vi "PH_VacuumControl.Search Device.vi"(0 "i ref in":refnum<vi>, 5 "error in (no error)":errorcluster) -> (14 "i ref out":refnum<vi>, 17 "Device found":bool, 19 "error out":errorcluster)   [LabVIEW 2014, in "PH_VacuumControl.lvlib"]
doc: "This VI searches for the device which is given by a firmware number. It is indicated if this is found succesfully, and connection data are written wo own attributes."
uses:
  PH_VacuumControl.lvlib
  instr.lib/AGCxxx/AGCxxx/AGCxxx VISA Control.ctl
  instr.lib/AGCxxx/AGCxxx - Driver.lvlib
  PH_Common/PH_Common.lvlib
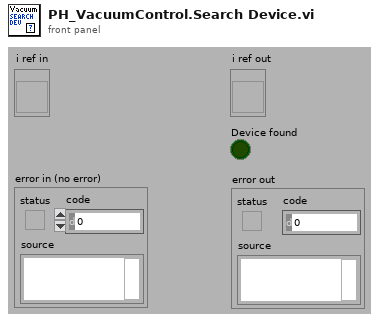
[diagram p1: front panel]
types:
  T1 = typedef "PH_VacuumControl.lvlib/PH_VacuumControl.i attribute.ctl" = cluster{"GUI Refs":cluster{"Exit":refnum<vi>, "Set Unit":refnum<vi>, "Device found":refnum<vi>, "Busy":refnum<vi>, "State":refnum<vi>, "Delete":refnum<vi>, "Channels":refnum<vi>, "Channel Name":refnum<vi>, "Trend":refnum<vi>, "Logarithmic":refnum<vi>, "Limit reached":refnum<vi>, "Channel Name 1 MT":refnum<vi>, "Channel Name 2 MT":refnum<vi>, "Trend MT":refnum<vi>, "Logarithmic MT":refnum<vi>, "Limit reached MT":refnum<vi>}, "Device found":bool, "Busy":bool, "Selected Unit":i32, "Channels [mbar]":T2, "Channel Names":cluster{"Channel 1":string, "Channel 2":string, "Channel 3":string, "Channel 4":string, "Channel 5":string, "Channel 6":string}, "Status":T3, "AGCxxx VISA Cluster":T4, "Instr Firmware Revision":string, "Service IDs Pressure":cluster{"Channel 1":i32, "Channel 2":i32, "Channel 3":i32, "Channel 4":i32, "Channel 5":i32, "Channel 6":i32}, "Service IDs Limits":cluster{"Channel 1":i32, "Channel 2":i32, "Channel 3":i32, "Channel 4":i32, "Channel 5":i32, "Channel 6":i32}, "Trend":cluster{"Start Point":timestamp, "Pressures [mbar] Channel 1":dbl[], "Pressures [mbar] Channel 2":dbl[], "Pressures [mbar] Channel 3":dbl[], "Pressures [mbar] Channel 4":dbl[], "Pressures [mbar] Channel 5":dbl[], "Pressures [mbar] Channel 6":dbl[], "Timebase [s]":i32[], "Trend Channel":u16, "Start Fit":dbl, "Trend Channel 1 MT":u16, "Trend Channel 2 MT":u16, "Start or continue Fit MT":dbl, "Continue or start Fit MT":dbl, "Datasets strored":i32, "Dataarray Size":i32}, "Running":bool}
  T2 = typedef "PH_VacuumControl.lvlib/PH_VacuumControl.Channels.ctl" = cluster{"Channel 1":dbl, "Channel 2":dbl, "Channel 3":dbl, "Channel 4":dbl, "Channel 5":dbl, "Channel 6":dbl, "Name Channel 1":string, "Name Channel 2":string, "Name Channel 3":string, "Name Channel 4":string, "Name Channel 5":string, "Name Channel 6":string, "Upper Limit":dbl, "Upper Limit 2":dbl, "Upper Limit 3":dbl, "Upper Limit 4":dbl, "Upper Limit 5":dbl, "Upper Limit 6":dbl}
  T3 = typedef "PH_StatusHandler.lvlib/PH_StatusHandler.Status.ctl" = i16
  T4 = typedef "AGCxxx - Driver.lvlib/AGCxxx VISA Control.ctl" = cluster{"VISA resource name":refnum<visa-resource-name>, "VISA Timeout Value (1000 ms)":u32, "Lock Timeout (1000 ms)":u32, "MAX Channel (6)":i32}
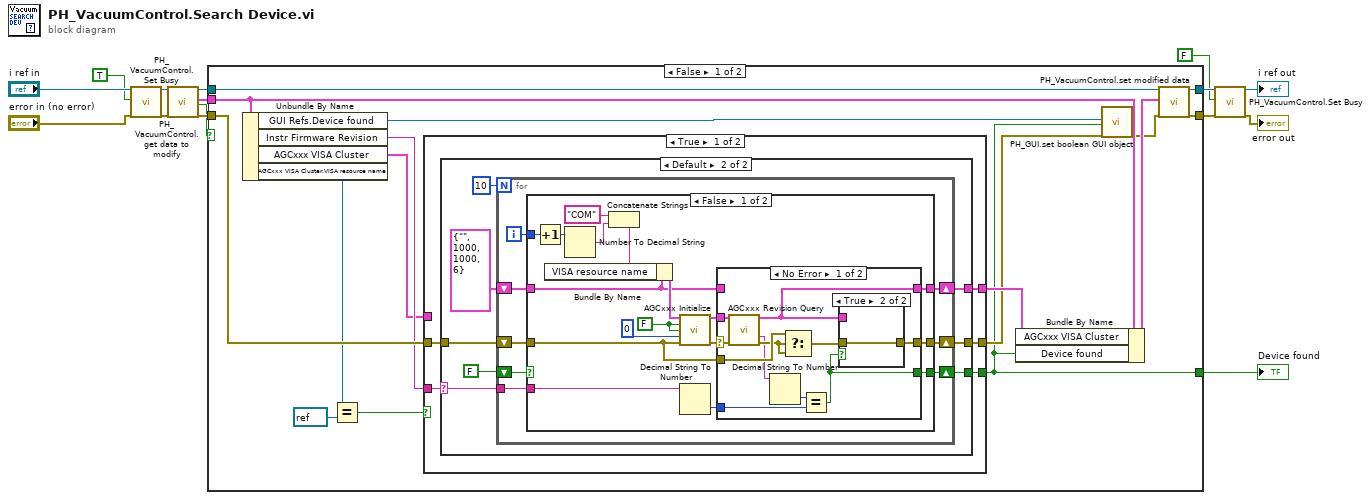
[diagram p0: block diagram]
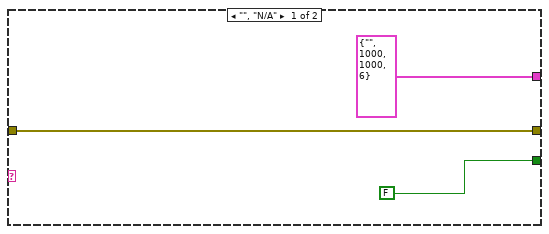
[diagram p2: hidden frame]
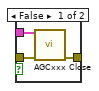
[diagram p3: hidden frame]
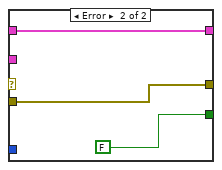
[diagram p4: hidden frame]
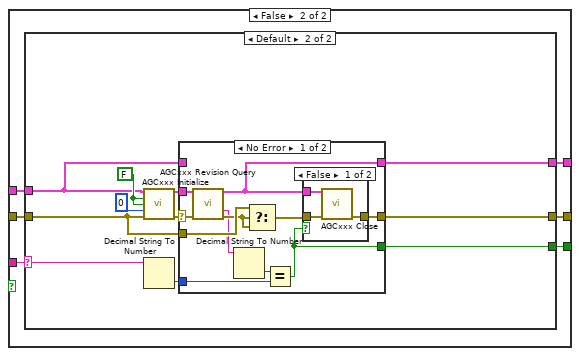
[diagram p6: hidden frame]
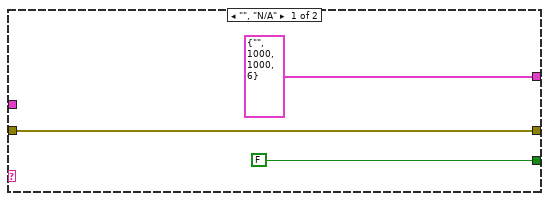
[diagram p7: hidden frame]
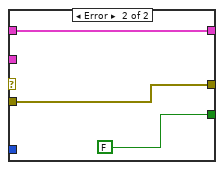
[diagram p9: hidden frame]
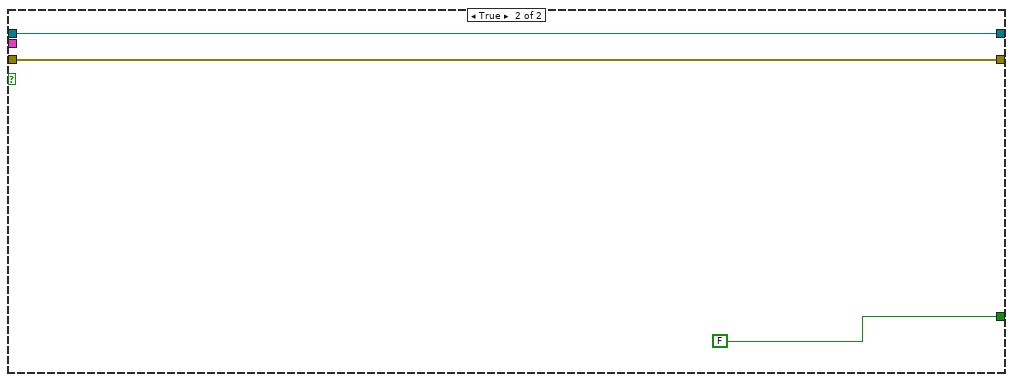
[diagram p10: hidden frame]
diagram:
  n1 = call "PH_VacuumControl.Set Busy.vi"("i ref in"="i ref in", "Busy"=TRUE, "error in (no error)"="error in (no error)") -> ("i ref out"=w7:refnum<vi>, "error out"=w9:errorcluster)  [unwired: 14 in, 1 out]
  n2 = call "PH_VacuumControl.get data to modify.vi"("i ref in"=w7, "error in (no error)"=w9) -> ("i ref out"=w14:refnum<vi>, "i attribute"=w13:T1, "timed out"=w12:bool, "error out"=w15:errorcluster)  [unwired: 14 in]
  n3 = case shown="False" w12 {
    tunnel: w15 -> [w31 w133]
    tunnel: w14 -> [w29 w134]
    tunnel: w13 -> [w28 _]
    tunnel: [w26 w133] -> w4
    tunnel: [w24 w134] -> w2
    tunnel: [w20 FALSE] -> w11
    frame False {
      n4 = Unbundle By Name(w28) -> ("GUI Refs.Device found"=w23:refnum<vi>, "Instr Firmware Revision"=w30:string, "AGCxxx VISA Cluster"=w16:T4, "AGCxxx VISA Cluster.VISA resource name"=w19:refnum<visa-resource-name>)
      n5 = Equal?(x=w19, y=refnum<visa-resource-name> refnum ("AGCxxx VISA Cluster.VISA resource name")) -> (x = y?=w17:bool)
      n6 = case shown="True" w17 {
        tunnel: w31 -> [w36 w99]
        tunnel: w30 -> [w35 w98]
        tunnel: [w34 w97] -> w27
        tunnel: [w33 w96] -> w22
        tunnel: [w32 w95] -> w20
        tunnel: w16 -> [_ w94]
        frame True {
          n7 = case shown="Default" w35 {
            selector: w35 -> [_ w43]
            tunnel: [FALSE w47] -> w32
            tunnel: [T4 {"VISA resource name"="", "VISA Timeout Value (1000 ms)"=1000, "Lock Timeout (1000 ms)"=1000, "MAX Channel (6)"=6} ("dup AGCxxx VISA Cluster") w46] -> w34
            tunnel: [w39 w45] -> w33
            tunnel: w36 -> [w39 w44]
            frame "", "N/A" {
            }
            frame Default {
              n8 = for {
                N: 10 -> [_]
                tunnel: w43 -> [w51]
                shift-right: [w53] -> w45
                shift-left: w44 -> [w52]
                shift-right: [w55] -> w47
                shift-left: FALSE -> [w49]
                shift-right: [w54] -> w46
                shift-left: T4 {"VISA resource name"="", "VISA Timeout Value (1000 ms)"=1000, "Lock Timeout (1000 ms)"=1000, "MAX Channel (6)"=6} ("dup AGCxxx VISA Cluster") -> [w48]
                i -> [w50]
                n9 = case shown="False" w49 {
                  selector: w49 -> [_ w91]
                  tunnel: [w71 w91] -> w55
                  tunnel: [w70 w93] -> w54
                  tunnel: [w69 w92] -> w53
                  tunnel: w52 -> [w59 w92]
                  tunnel: w51 -> [w57 _]
                  tunnel: w50 -> [w63 _]
                  tunnel: w48 -> [w58 w93]
                  frame False {
                    w66 = FALSE ("ID Query (T: Check)")
                    n10 = Increment(x=w63) -> (x+1=w62:i32)
                    n11 = Number To Decimal String(number=w62) -> (decimal integer string=w61:string)  [unwired: 1 in]
                    n12 = Concatenate Strings("COM", w61) -> (w64:string)
                    n13 = Bundle By Name(cluster=w58, "VISA resource name"=w64) -> (w72:T4)
                    n14 = call "AGCxxx Initialize.vi"("AGCxxx VISA Cluster"=w72, "ID Query (T: Check)"=w66, "Reset (T: Reset)"=w66, "access mode"=u32 0, "error in (no error)"=w59) -> ("dup AGCxxx VISA Cluster"=w68:T4, "error out"=w60:errorcluster)  [unwired: 9 in]
                    n15 = Decimal String To Number(string=w57) -> (number=w56:i32)  [unwired: 2 in, 1 out]
                    n16 = case shown="No Error" w60 {
                      selector: w60 -> [w78 _]
                      tunnel: [w83 FALSE] -> w71
                      tunnel: [w82 w89] -> w70
                      tunnel: [w81 w90] -> w69
                      tunnel: w68 -> [w80 _]
                      tunnel: w56 -> [w79 _]
                      tunnel: w59 -> [w76 w90]
                      tunnel: w58 -> [_ w89]
                      frame No Error {
                        n17 = call "AGCxxx Revision Query.vi"("AGCxxx VISA Cluster"=w80, "error in (no error)"=w78) -> ("dup AGCxxx VISA Cluster"=w82:T4, "Instr Firmware Revision"=w74:string, "error out"=w75:errorcluster)  [unwired: 10 in, 1 out]
                        n18 = Decimal String To Number(string=w74) -> (number=w73:i32)  [unwired: 2 in, 1 out]
                        n19 = Select(t=w76, s=w75, f=w75) -> (s? t:f=w77:errorcluster)
                        n20 = Equal?(x=w73, y=w79) -> (x = y?=w83:bool)
                        n21 = case shown="True" w83 {
                          tunnel: [w86 w87] -> w81
                          tunnel: w82 -> [w85 _]
                          tunnel: w77 -> [w84 w87]
                          frame False {
                            n22 = call "AGCxxx Close.vi"("AGCxxx VISA Cluster"=w85, "error in (no error)"=w84) -> ("error out"=w86:errorcluster)  [unwired: 13 in]
                          }
                          frame True {
                          }
                        }
                      }
                      frame Error {
                      }
                    }
                  }
                  frame True {
                  }
                }
              }
            }
          }
        }
        frame False {
          n23 = case shown="Default" w98 {
            selector: w98 -> [_ w109]
            tunnel: [FALSE w113] -> w95
            tunnel: [T4 {"VISA resource name"="", "VISA Timeout Value (1000 ms)"=1000, "Lock Timeout (1000 ms)"=1000, "MAX Channel (6)"=6} ("dup AGCxxx VISA Cluster") w112] -> w97
            tunnel: [w102 w111] -> w96
            tunnel: w99 -> [w102 w110]
            tunnel: w94 -> [_ w103]
            frame "", "N/A" {
            }
            frame Default {
              w106 = FALSE ("ID Query (T: Check)")
              n24 = call "AGCxxx Initialize.vi"("AGCxxx VISA Cluster"=w103, "ID Query (T: Check)"=w106, "Reset (T: Reset)"=w106, "access mode"=u32 0, "error in (no error)"=w110) -> ("dup AGCxxx VISA Cluster"=w108:T4, "error out"=w105:errorcluster)  [unwired: 9 in]
              n25 = Decimal String To Number(string=w109) -> (number=w104:i32)  [unwired: 2 in, 1 out]
              n26 = case shown="No Error" w105 {
                selector: w105 -> [w119 _]
                tunnel: [w124 FALSE] -> w113
                tunnel: [w123 w129] -> w112
                tunnel: [w122 w131] -> w111
                tunnel: w108 -> [w121 _]
                tunnel: w104 -> [w120 _]
                tunnel: w110 -> [w117 w131]
                tunnel: w103 -> [_ w129]
                frame No Error {
                  n27 = call "AGCxxx Revision Query.vi"("AGCxxx VISA Cluster"=w121, "error in (no error)"=w119) -> ("dup AGCxxx VISA Cluster"=w123:T4, "Instr Firmware Revision"=w115:string, "error out"=w116:errorcluster)  [unwired: 10 in, 1 out]
                  n28 = Decimal String To Number(string=w115) -> (number=w114:i32)  [unwired: 2 in, 1 out]
                  n29 = Select(t=w117, s=w116, f=w116) -> (s? t:f=w118:errorcluster)
                  n30 = Equal?(x=w114, y=w120) -> (x = y?=w124:bool)
                  n31 = case shown="False" w124 {
                    tunnel: [w127 w128] -> w122
                    tunnel: w123 -> [w126 _]
                    tunnel: w118 -> [w125 w128]
                    frame False {
                      n32 = call "AGCxxx Close.vi"("AGCxxx VISA Cluster"=w126, "error in (no error)"=w125) -> ("error out"=w127:errorcluster)  [unwired: 13 in]
                    }
                    frame True {
                    }
                  }
                }
                frame Error {
                }
              }
            }
          }
        }
      }
      n33 = Bundle By Name(cluster=w28, "AGCxxx VISA Cluster"=w27, "Device found"=w20) -> (w25:T1)
      n34 = call "PH_GUI.set boolean GUI object.vi"("Boolean Knob GUI Ref"=w23, "Value"=w20, "error in (no error)"=w22) -> ("error out"=w21:errorcluster)  [unwired: 16 in]
      n35 = call "PH_VacuumControl.set modified data.vi"("i ref in"=w29, "i attribute"=w25, "error in (no error)"=w21) -> ("i ref out"=w24:refnum<vi>, "error out"=w26:errorcluster)  [unwired: 15 in]
    }
    frame True {
    }
  }
  "Device found" <- w11
  n36 = call "PH_VacuumControl.Set Busy.vi"("i ref in"=w2, "Busy"=FALSE, "error in (no error)"=w4) -> ("i ref out"=→"i ref out":refnum<vi>, "error out"=→"error out":errorcluster)  [unwired: 14 in, 1 out]
